vi "Read FrameHeight 2.vi"(8 "error in (no error)":errorcluster, 11 "Kinect Session in":refnum<class "Kinect Session.lvclass">) -> (0 "error out":errorcluster, 2 "FrameHeight":i32, 3 "Kinect Session out":refnum<class "Kinect Session.lvclass">)   [LabVIEW 2011, in "Kinect Session.lvclass"]
uses:
  Kinect Session.lvclass
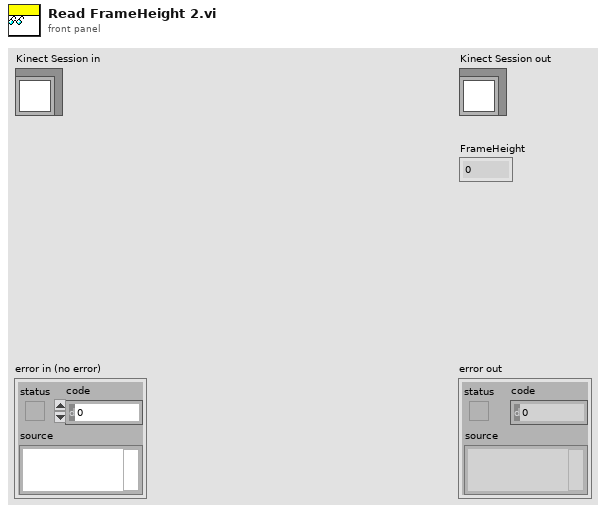
[diagram p1: front panel]
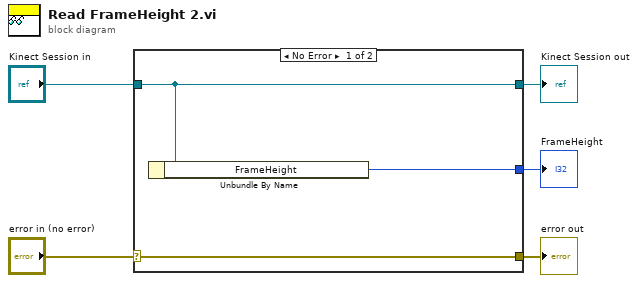
[diagram p0: block diagram]
diagram:
  n1 = case shown="No Error" "error in (no error)" {
    selector: "error in (no error)" -> [w8 w9]
    tunnel: [w8 w9] -> w4
    tunnel: [w7 w10] -> w2
    tunnel: "Kinect Session in" -> [w7 w10]
    tunnel: [w6 _] -> w1
    frame No Error {
      n2 = Unbundle By Name(w7) -> ("FrameHeight"=w6:i32)
    }
    frame Error {
    }
  }
  "error out" <- w4
  "Kinect Session out" <- w2
  "FrameHeight" <- w1
